vi "Keithley Max_P List_IIT.vi"(0 "VISA resource name in":refnum<visa-resource-name>, 7 "t=0 timestamp":sgl, 9 "Light?":bool, 11 "Voltage List":dbl[](array[numeric])) -> (4 "VISA resource name out":refnum<visa-resource-name>, 6 "Data Array":dbl[][](array[numeric]), 8 "timestamp":sgl, 15 "Measurement Complete":bool)   [LabVIEW 2016]
doc: "Configures a sweep and takes voltage and current readings at each point."
uses:
  C:/Program Files (x86)/National Instruments/LabVIEW 2016/instr.lib/keithley_24xx/Keithley 24XX/Public/Data/Read (Multiple Points).vi
  C:/Program Files (x86)/National Instruments/LabVIEW 2016/instr.lib/keithley_24xx/Keithley 24XX/Keithley 24XX.lvlib
panel:
  in  "Source Mode  (0: Voltage)":u16(ring) items=["Voltage", "Current"]
  # "(c) 2006 National Instruments.  ALL RIGHTS RESERVED."
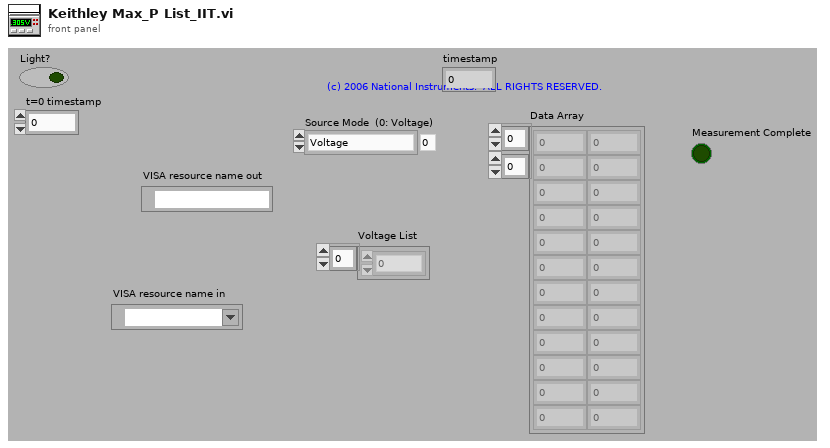
[diagram p1: front panel]
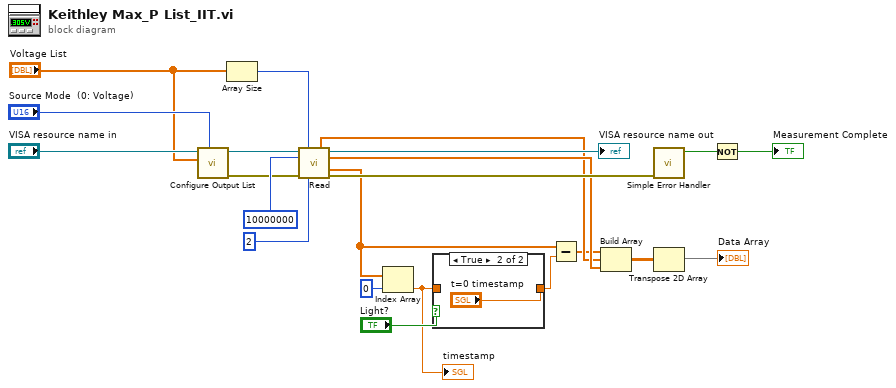
[diagram p0: block diagram]
diagram:
  n1 = call "Configure Output List.vi"("Source Mode  (0: Voltage)"="Source Mode  (0: Voltage)", "Output List"="Voltage List", "VISA resource name"="VISA resource name in") -> ("error out"=w15:errorcluster, "VISA resource name out"=w16:refnum<visa-resource-name>)  [unwired: 7 in]
  n2 = Array Size(array="Voltage List") -> (size(s)=w10:i32)
  n3 = call-poly "Read.vi"("VISA resource name"=w16, "Sample Count (1)"=w10, "Timeout (10000 ms)"=10000000, "error in (no error)"=w15, "Output Mode (0: Fixed)"=2) -> ("Voltage"=w9:sgl[], "VISA resource name out"=→"VISA resource name out":refnum<visa-resource-name>, "Current"=w12:sgl[], "Timestamp"=w7:sgl[], "error out"=w22:errorcluster)  [unwired: 4 in, 2 out]
  n4 = Index Array(array=w7, index=0) -> (element=w3:sgl)
  "timestamp" <- w3
  n5 = case shown="True" "Light?" {
    tunnel: [w23 "t=0 timestamp"] -> w4
    tunnel: w3 -> [w23 _]
    frame False {
    }
    frame True {
    }
  }
  n6 = Subtract(x=w7, y=w4) -> (x-y=w8:sgl[])
  n7 = Build Array(w8, w9, w12) -> (w2:sgl[][])
  n8 = call <vilib>:"Simple Error Handler.vi"("error in (no error)"=w22) -> ("error?"=w20:bool)  [unwired: 4 in, 4 out]
  n9 = Transpose 2D Array(2D array=w2) -> (transposed array=→"Data Array":sgl[][])
  n10 = Not(x=w20) -> (.not. x?=→"Measurement Complete":bool)
